vi "Extract_ROI_Image.vi"(4 "Dllindex":i32, 6 "CreatDllImage":bool, 8 "error in (no error)":errorcluster, 9 "Coordinate System Out":T3 {"Measurement System"."Axis Reference" items=["Direct", "Indirect"]; "Measurement System"."Angle (deg)" format="%.2f"; "Measurement System"."Origin"."Y" format="%.2f"; "Measurement System"."Origin"."X" format="%.2f"; "Reference System"."Axis Reference" items=["Direct", "Indirect"]; "Reference System"."Angle (deg)" format="%.2f"; "Reference System"."Origin"."Y" format="%.2f"; "Reference System"."Origin"."X" format="%.2f"}, 10 "ROI Entry":T4={"vROIName"="", "vROIContour"={"Contour Type"=0, "ROI Type"=0, "Points"=[]}, "ProcessSetting"=[], "Analysis_Setting"={"PreProcess"=enum."*Algorithm*", "Parameter"=""}}, 11 "ImageIn":T1(plugin-control)) -> (0 "error out":errorcluster, 2 "ForCalCalculaton Out":T1, 3 "ExtractedOriginalImage":T1(plugin-control))   [LabVIEW 2019]
uses:
  <vilib>/vision/NI_Vision_Development_Module.lvlib
  DLL/[Global] ExtractedImage.vi
  DLL/[Global]ForCalCalculaton.vi
  Analysis/Controls/Analysis_Setting.ctl
  Process/Controls/Process_Setting.ctl
  Controls/Vision_DataEntry.ctl
  <vilib>/vision/Image Controls.llb/IMAQ Image.ctl
  Ctrl/VisionProcessName.ctl
panel:
  out "ROI Descriptor out":T2 {"Contours"."Type" items=["No Selection", "Point", "Line", "Rectangle", "Oval", "Polygon", "Freehand Region", "Annulus", "Unused2", "Unused3", "Broken Line", "Freehand Line", "Rotated Rectangle"]}
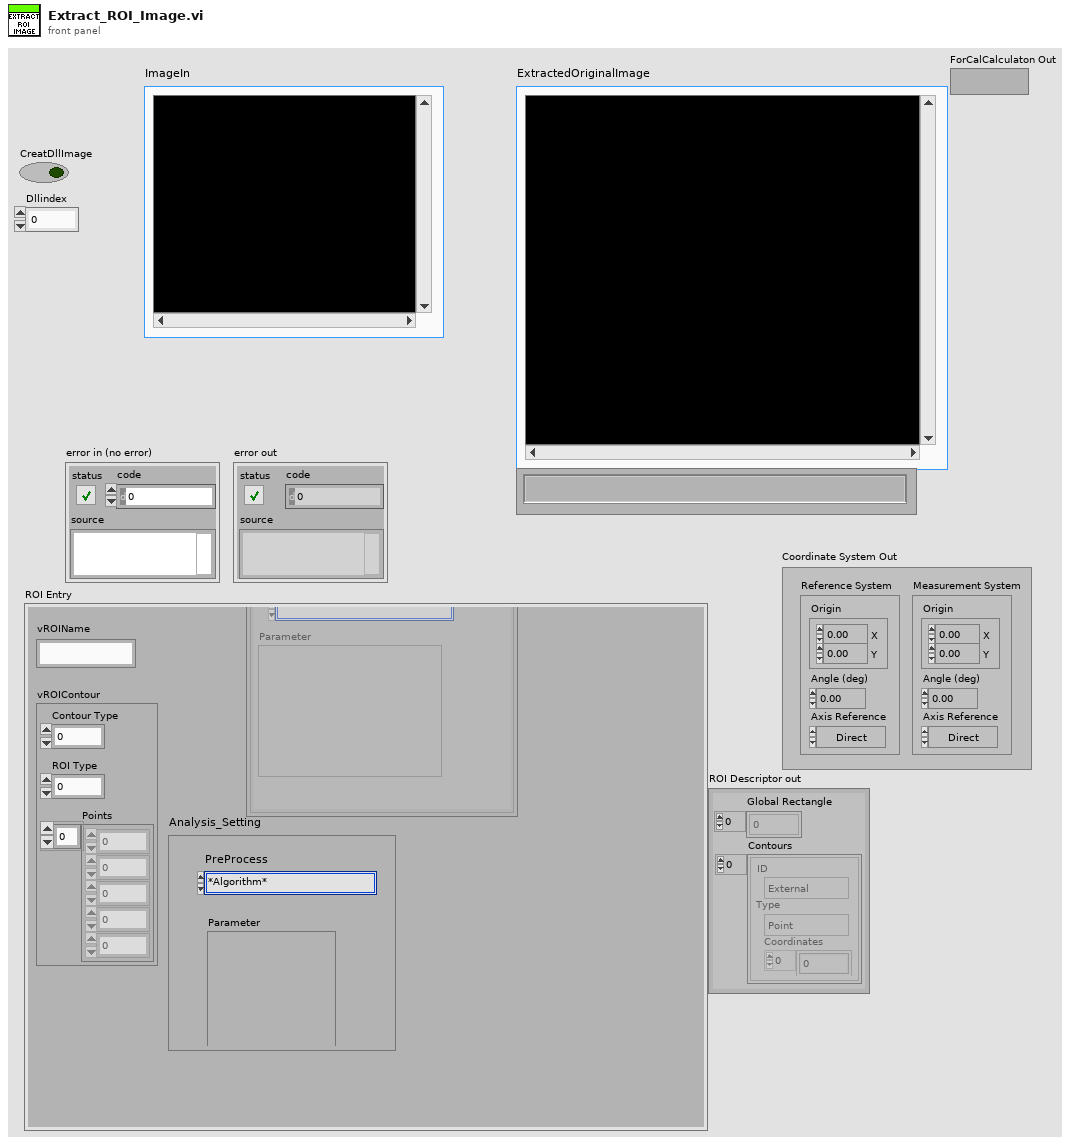
[diagram p1: front panel]
types:
  T1 = typedef "IMAQ Image.ctl" = refnum<image>
  T2 = typedef "ROI Descriptor" = cluster{"Global Rectangle":i32[], "Contours":cluster{"ID":enum32{"External", "Internal"}, "Type":u32, "Coordinates":i32[]}[]}
  T3 = typedef "IMAQ Coordinate System" = cluster{"Reference System":cluster{"Origin":cluster{"X":sgl, "Y":sgl}, "Angle (deg)":sgl, "Axis Reference":u32}, "Measurement System":cluster{"Origin":cluster{"X":sgl, "Y":sgl}, "Angle (deg)":sgl, "Axis Reference":u32}}
  T4 = typedef "Vision_DataEntry.ctl" = cluster{"vROIName":string, "vROIContour":cluster{"Contour Type":u32, "ROI Type":u32, "Points":i32[]}, "ProcessSetting":T5[], "Analysis_Setting":T7}
  T5 = typedef "Process_Setting.ctl" = cluster{"Enum_PreProcess":T6, "Parameter":string}
  T6 = typedef "VisionProcessName.ctl" = enum16{"*CamParameter*", "CamAttributes", "*Preprocess*", "CG_Brightness", "C_Plane Extraction", "C_Threshold", "G_Lookup Table", "G_Threshold"}
  T7 = typedef "Analysis_Setting.ctl" = cluster{"PreProcess":T8, "Parameter":string}
  T8 = typedef "VisionProcessName.ctl" = enum16{"*CamParameter*", "CamAttributes", "*Preprocess*", "CG_Brightness", "C_Plane Extraction", "C_Threshold", "G_Lookup Table", "G_Threshold", "B_Image Inversion", "*Algorithm*", "CG_Histogram", "C_Color Matching", "C_Color Pattern Matching", "G_PatternMatch", "CG_Find Straight Edge", "CG_Adv. Find Straight Edge", "CG_Find Circular Edge", "G_Max Clamp", "G_Clamp (Rake)", "G_Pattern Matching"}
  T9 = typedef "Image Type" = u32
  T10 = cluster{"Origin":cluster{"X":sgl, "Y":sgl}, "Angle (deg)":sgl, "Axis Reference":u32}
  T11 = cluster{"Contour Type":u32, "ROI Type":u32, "Points":i32[]}
  T12 = cluster{"Contour Type":u32, "ROI Type":u32, "Points":i32[]}[]
  T13 = cluster{"Points":i32[], cluster{"Contour Type":u32, "ROI Type":u32, "Points":i32[]}[]}
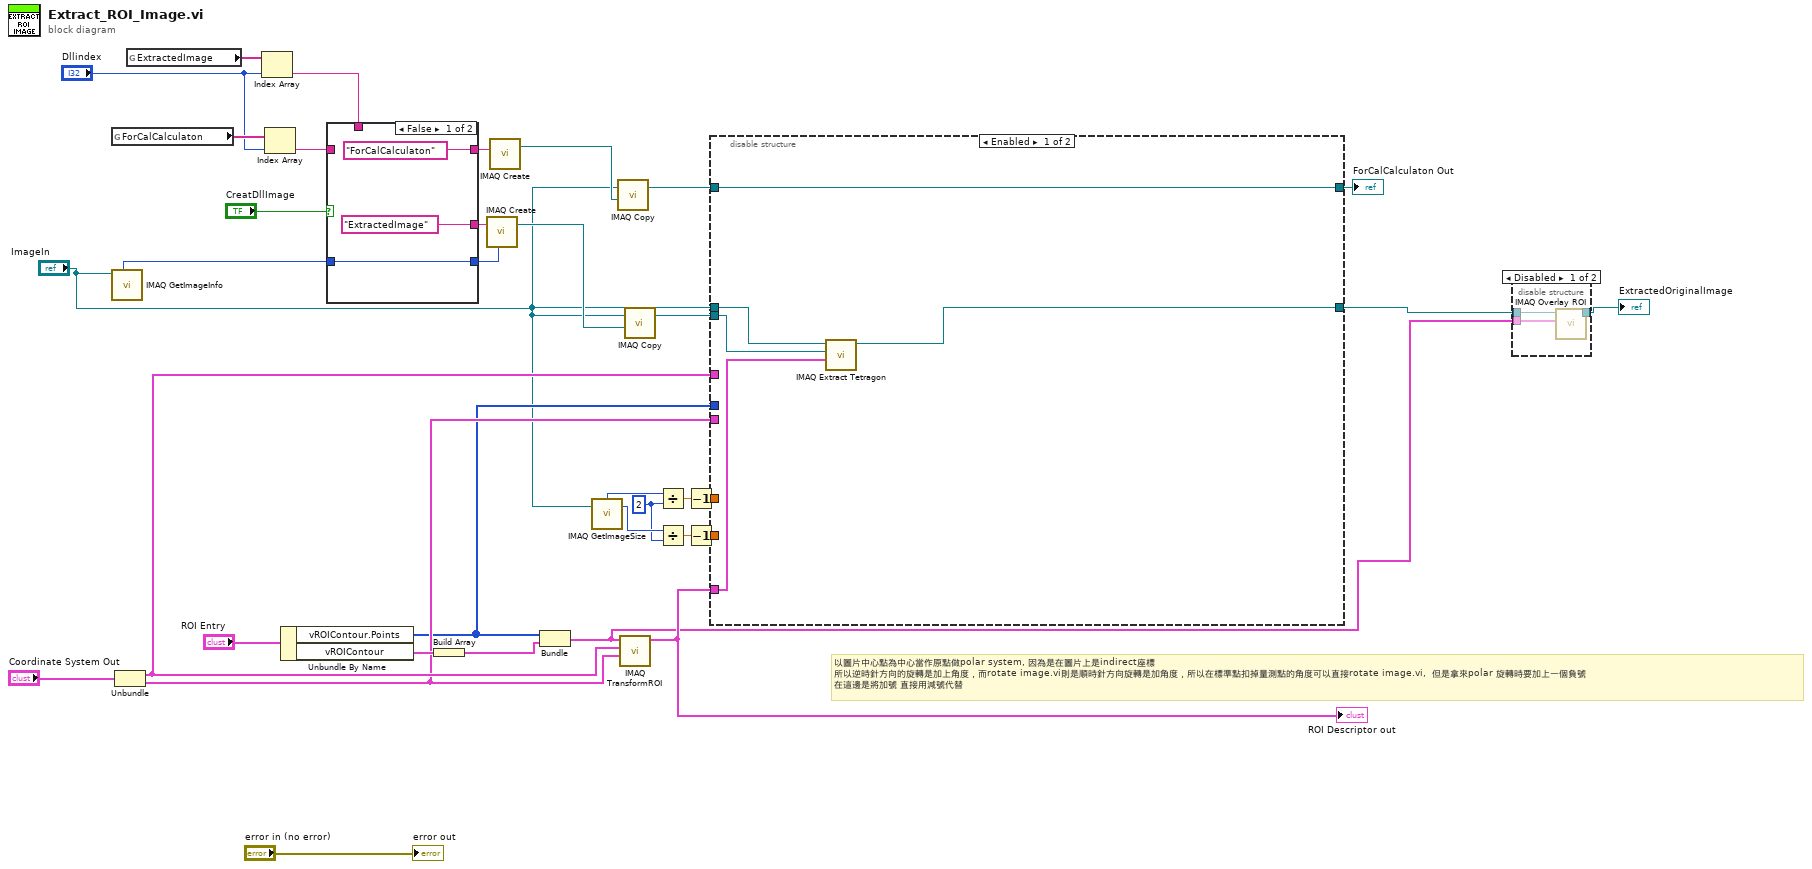
[diagram p0: block diagram]
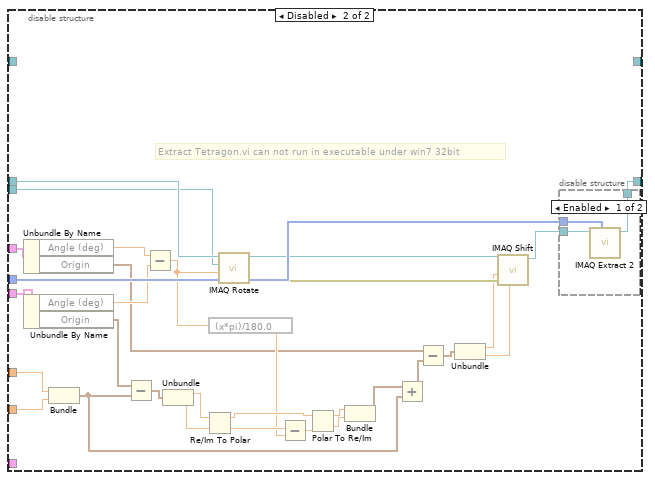
[diagram p4: hidden frame]
diagram:
  w20 = 2 ("y")
  # "以圖片中心點為中心當作原點做polar system, 因為是在圖片上是indirect座標\n所以逆時針方向的旋轉是加上角度，而rotate image.vi則是順時針方向旋轉是加角度，所以在標準點扣掉量測點的角度可以直接rotate image.vi,  但是拿來polar 旋轉時要加上一個負號\n在這邊是將加號 直接用減號代替"
  n1 = global read "[Global]ForCalCalculaton.vi" "ForCalCalculaton"() -> (w4:string[])
  n2 = call "IMAQ GetImageInfo"("Image"="ImageIn") -> ("Image Type"=w35:T9)  [unwired: 3 in, 7 out]
  n3 = Unbundle("Coordinate System Out") -> ("Reference System"=w28:T10, "Measurement System"=w27:T10)
  n4 = global read "[Global] ExtractedImage.vi" "ExtractedImage"() -> (w14:string[])
  n5 = Index Array(array=w14, index="Dllindex") -> (element=w13:string)
  n6 = Index Array(array=w4, index="Dllindex") -> (element=w2:string)
  n7 = Unbundle By Name("ROI Entry") -> ("vROIContour.Points"=w26:i32[], "vROIContour"=w32:T11)
  n8 = case shown="False" "CreatDllImage" {
    tunnel: w35 -> [w37 w40]
    tunnel: w13 -> [_ w41]
    tunnel: ["ExtractedImage" ("Image Name") w41] -> w12
    tunnel: [w37 w40] -> w11
    tunnel: ["ForCalCalculaton" ("Image Name") w39] -> w8
    tunnel: w2 -> [_ w39]
    frame False {
    }
    frame True {
      # "Add for dll"
    }
  }
  n9 = Build Array(w32) -> (w31:T12)
  n10 = call "IMAQ Create"("Image Name"=w12, "Image Type"=w11) -> ("New Image"=w9:T1)  [unwired: 2 in, 2 out]
  n11 = call "IMAQ Create"("Image Name"=w8) -> ("New Image"=w5:T1)  [unwired: 3 in, 2 out]
  n12 = Bundle("Points"=w26, w31) -> (w23:T13)  [unwired: 1 in]
  n13 = call "IMAQ GetImageSize"("Image"="ImageIn") -> ("Y Resolution"=w21:i32, "X Resolution"=w22:i32)  [unwired: 3 in, 1 out]
  n14 = call "IMAQ Copy"("Image Dst"=w5, "Image Src"="ImageIn") -> ("Image Dst Out"=w7:T1)  [unwired: 4 in, 1 out]
  n15 = call "IMAQ TransformROI"("New Reference"=w27, "Base Reference"=w28, "ROI Descriptor"=w23) -> ("ROI Descriptor out"=w30:T2)  [unwired: 7 in, 1 out]
  "ROI Descriptor out" <- w30
  n16 = call "IMAQ Copy"("Image Dst"=w9, "Image Src"="ImageIn") -> ("Image Dst Out"=w10:T1)  [unwired: 4 in, 1 out]
  n17 = Divide(x=w22, y=w20) -> (x/y=w19:dbl)
  n18 = Divide(x=w21, y=w20) -> (x/y=w18:dbl)
  n19 = Decrement(x=w19) -> (x-1=w17:dbl)
  n20 = Decrement(x=w18) -> (x-1=w16:dbl)
  n21 = disable-structure shown="Enabled" {
    disable-tunnel: "ImageIn" -> [w46 w76]
    disable-tunnel: w10 -> [w45 w73]
    disable-tunnel: [w44 w74] -> w25
    disable-tunnel: w30 -> [w43 _]
    disable-tunnel: w28 -> [_ w77]
    disable-tunnel: w27 -> [_ w68]
    disable-tunnel: w26 -> [_ w75]
    disable-tunnel: w17 -> [_ w59]
    disable-tunnel: w16 -> [_ w58]
    disable-tunnel: [w42 _] -> w6
    disable-tunnel: w7 -> [w42 _]
    frame Enabled {
      n22 = call-poly "IMAQ Extract Tetragon"("ROI Descriptor"=w43, "Image Dst"=w45, "Image Src"=w46) -> ("Image Dst Out"=w44:T1)  [unwired: 7 in, 1 out]
    }
    frame Disabled {
      # "Extract Tetragon.vi can not run in executable under win7 32bit"
      n23 = Unbundle By Name(w77) -> ("Angle (deg)"=w72:sgl, "Origin"=w48:cluster{"X":sgl, "Y":sgl})
      n24 = Unbundle By Name(w68) -> ("Angle (deg)"=w67:sgl, "Origin"=w54:cluster{"X":sgl, "Y":sgl})
      n25 = Bundle(w59, w58) -> (w52:cluster{dbl, dbl})  [unwired: 1 in]
      n26 = Subtract(x=w54, y=w52) -> (x-y=w57:cluster{dbl, dbl})
      n27 = Subtract(x=w72, y=w67) -> (x-y=w60:sgl)
      n28 = Unbundle(w57) -> (w56:dbl, w55:dbl)
      n29 = Re/Im To Polar(2:w55, 3:w56) -> (0:w51:dbl, 1:w66:dbl)
      n30 = expression code="(x*pi)/180.0" ("radians to degrees")(w60) -> (w50:sgl)
      n31 = call "IMAQ Rotate"("Angle (degrees)"=w60, "Image Dst"=w73, "Image Src"=w76) -> ("error out"=w71:errorcluster, "Image Dst Out"=w70:T1)  [unwired: 7 in]
      n32 = Subtract(x=w51, y=w50) -> (x-y=w49:dbl)
      n33 = Polar To Re/Im(2:w49, 3:w66) -> (0:w64:dbl, 1:w65:dbl)
      n34 = Bundle(w65, w64) -> (w53:cluster{dbl, dbl})  [unwired: 1 in]
      n35 = Add(x=w53, y=w52) -> (x+y=w47:cluster{dbl, dbl})
      n36 = Subtract(x=w48, y=w47) -> (x-y=w63:cluster{dbl, dbl})
      n37 = Unbundle(w63) -> (w62:dbl, w61:dbl)
      n38 = call "IMAQ Shift"("YOffset"=w61, "error in (no error)"=w71, "XOffset"=w62, "Image Src"=w70) -> ("Image Dst Out"=w69:T1)  [unwired: 6 in, 1 out]
      n39 = disable-structure shown="Enabled" {
        disable-tunnel: w69 -> [w80 w81]
        disable-tunnel: w75 -> [w79 _]
        disable-tunnel: [w78 w81] -> w74
        frame Enabled {
          n40 = call "IMAQ Extract 2"("Optional Rectangle"=w79, "Image Src"=w80) -> ("Image Dst Out"=w78:T1)  [unwired: 8 in, 1 out]
        }
        frame Disabled {
        }
      }
    }
  }
  "ForCalCalculaton Out" <- w6
  n41 = disable-structure shown="Disabled" {
    disable-tunnel: w25 -> [w84 w85]
    disable-tunnel: [w83 w85] -> w24
    disable-tunnel: w23 -> [w82 _]
    frame Disabled {
      n42 = call "IMAQ Overlay ROI"("ROI Descriptor"=w82, "Image"=w84) -> ("Image Out"=w83:T1)  [unwired: 8 in, 1 out]
    }
    frame Enabled {
    }
  }
  "ExtractedOriginalImage" <- w24
  "error out" <- "error in (no error)"
